vi "Write Config Value.vi"(2 "error in (no error)":errorcluster, 3 "Value":dbl format="%.2f", 4 "Key":string, 5 "input cluster":T1 {"MaxLambdaCurrent [A]" format="%.2f"; "LambdaRates [A/min]" format="%.2f"; "MaxNormalCurrent [A]" format="%.2f"; "StabilitySetting [%]" format="%.2f"; "FieldCurrentRatio [T/A]" format="%.2f"; "SwitchWaitTime [s]" format="%.2f"; "SwitchHtrCurrent [mA]" format="%.2f"; "TrainRates [A/min]" format="%.2f"; "NormalRates [A/min]" format="%.2f"; "Breakpts [A]" format="%.2f"}) -> (0 "error out":errorcluster, 1 "message":string=" INSTRUCTIONS:\r\rNormal Use:  When using subVIs that incorporate the error in/error out (or error I/O) structure, place this handler where you want to inform the user of an error, typically at the end of the I/O data path, as the last action of the program.  If the error in error? is ERROR, the handler creates a message describing the error and its source.  If the type of dialog = 1 (default), the message is displayed to the user, who can only acknowedge it.  If the type = 2, the user can acknowledge the message or abort execution; aborting a program with active I/O is not recommended.  If the type = 0, no message is displayed; this is used to process the error programmatically, and the error out cluster elements are wired to individual terminals for that reason.  \r\rOther Use:\n\r\nlocal testing.  To test the error code of a subVI or function that does not have the error I/O structure, you can wire its error code and a source string to the local error code and error source inputs.  If error in error? indicates no error and error code is not equal to 0, the local code and source are substituted for the error in values, and error? is set TRUE (ERROR).")   [LabVIEW 2021]
uses:
  <vilib>/Utility/config.llb/Write Key (String).vi
  <vilib>/Utility/config.llb/NI_LVConfig.lvlib
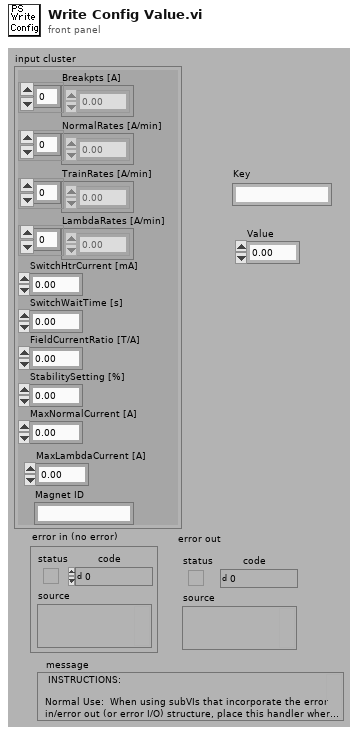
[diagram p1: front panel]
types:
  T1 = cluster{"Breakpts [A]":dbl[], "NormalRates [A/min]":dbl[], "TrainRates [A/min]":dbl[], "SwitchHtrCurrent [mA]":dbl, "SwitchWaitTime [s]":dbl, "FieldCurrentRatio [T/A]":dbl, "StabilitySetting [%]":dbl, "MaxNormalCurrent [A]":dbl, "Magnet ID":string, "LambdaRates [A/min]":dbl[], "MaxLambdaCurrent [A]":dbl}
  T2 = typedef "NI_LVConfig.lvlib/Config Data RefNum.ctl" = refnum<k1>
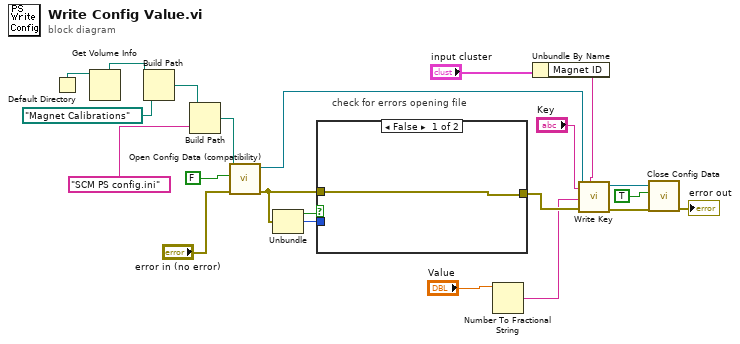
[diagram p0: block diagram]
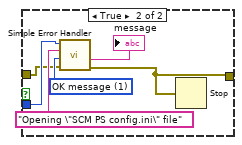
[diagram p2: hidden frame]
diagram:
  # "check for errors opening file"
  n1 = Default Directory() -> (w18:path)
  n2 = Get Volume Info(11:w18) -> (5:w16:path)  [unwired: 1 in, 5 out]
  n3 = Build Path(base path=w16, name or relative path=path "Magnet Calibrations") -> (appended path=w19:path)
  n4 = Build Path(base path=w19, name or relative path="SCM PS config.ini") -> (appended path=w12:path)
  n5 = call <vilib>:"Open Config Data (compatibility).vi"("error in (no error)"="error in (no error)", "create file if necessary (T)"=FALSE ("create file if necessary? (T)"), "configuration file path"=w12) -> ("error out"=w13:errorcluster, "refnum"=w10:T2)  [unwired: 6 in, 1 out]
  n6 = Unbundle(w13) -> ("status"=w15:bool, "code"=w14:i32)  [unwired: 1 out]
  n7 = case shown="False" w15 {
    tunnel: w14 -> [_ w29]
    tunnel: w13 -> [w23 w25]
    tunnel: [w23 w24] -> w11
    frame False {
    }
    frame True {
      w26 = u16 1 items=["no dialog", "OK message", "continue or stop message"] ("type of dialog (OK msg:1)")
      n8 = call <vilib>:"Simple Error Handler.vi"("error code (no error:0)"=w29, "error source (\" \")"="Opening \"SCM PS config.ini\" file" ("error source (\" \")"), "type of dialog (OK msg:1)"=w26, "error in (no error)"=w25) -> ("source out"=→"message":string, "error out"=w24:errorcluster)  [unwired: 1 in, 3 out]
      n9 = Stop(stop? (T)=w24) -> ()
    }
  }
  n10 = Number To Fractional String(number="Value") -> (F-format string=w7:string)  [unwired: 3 in]
  n11 = Unbundle By Name("input cluster") -> ("Magnet ID"=w1:string)
  n12 = call-poly <vilib>:"Write Key.vi"("section"=w1, "error in (no error)"=w11, "value"=w7, "key"="Key", "refnum"=w10) -> ("error out"=w6:errorcluster, "refnum out"=w5:T2)  [unwired: 4 in, 1 out]
  n13 = call <vilib>:"Close Config Data.vi"("error in (no error)"=w6, "write file if changed (T)"=TRUE ("write configuration file? (F)"), "refnum"=w5) -> ("error out"=→"error out":errorcluster)  [unwired: 7 in, 1 out]
